vi "Send Settings.vi"(8 "error in":errorcluster, 11 "6700 in":refnum<class "6700.lvclass">) -> (0 "error out":errorcluster, 3 "6700 out":refnum<class "6700.lvclass">)   [LabVIEW 2018, in "6700.lvlib" / "6700.lvclass"]
uses:
  6700.lvclass
  6700.lvclass/6700.ctl
  <instrlib>/Agilent N6700 Series/Agilent N6700 Series.lvlib
  builds/Power_Supply.lvlibp/Power Supply.lvclass
  C:/Users/Ron.Dexter.LUMINARTECH/Desktop/builds/Power_Supply.lvlibp/Power Supply.lvclass
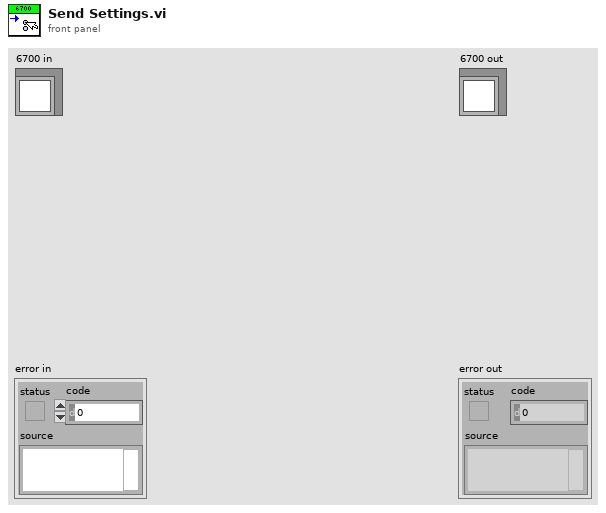
[diagram p1: front panel]
types:
  T1 = typedef "Power_Supply.lvlibp/Supply Settings.ctl" = cluster{"Voltage":dbl, "Current":dbl, "Output":bool}
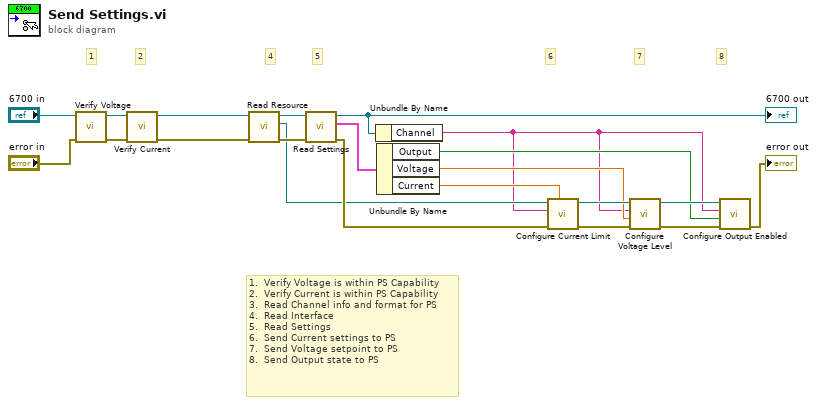
[diagram p0: block diagram]
diagram:
  # "1.  Verify Voltage is within PS Capability\n2.  Verify Current is within PS Capability\n3.  Read Channel info and format for PS\n4.  Read Interface\n5.  Read Settings\n6.  Send Current settings to PS\n7.  Send Voltage setpoint to PS\n8.  Send Output state to PS"
  # "8"
  # "7"
  # "6"
  # "5"
  # "4"
  # "2"
  # "1"
  n1 = call "Verify Voltage.vi"("error in"="error in", "6700 in"="6700 in") -> ("error out"=w19:errorcluster, "6700 out"=w21:refnum<class "6700.lvclass">)  [unwired: 8 in]
  n2 = call "Verify Current.vi"("error in"=w19, "6700 in"=w21) -> ("error out"=w4:errorcluster, "6700 out"=w3:refnum<class "6700.lvclass">)  [unwired: 8 in]
  n3 = call "Read Resource.vi"("error in"=w4, "Power Supply in"=w3) -> ("error out"=w6:errorcluster, "Resource"=w5:refnum<visa-resource-name>, "Power Supply out"=w7:refnum<class "6700.lvclass">)  [unwired: 7 in]
  n4 = call "Read Settings.vi"("error in (no error)"=w6, "Power Supply in"=w7) -> ("error out"=w11:errorcluster, "Settings"=w12:T1, "Power Supply out"=w1:refnum<class "6700.lvclass">)  [unwired: 7 in]
  "6700 out" <- w1
  n5 = Unbundle By Name(w1) -> ("Channel"=w2:string)
  n6 = Unbundle By Name(w12) -> ("Output"=w8:bool, "Voltage"=w9:dbl, "Current"=w10:dbl)
  n7 = call <instrlib>:"Configure Current Limit.vi"("Limit (0.0 amps)"=w10, "error in (no error)"=w11, "Channel Name (1)"=w2, "VISA resource name"=w5) -> ("error out"=w15:errorcluster, "VISA resource name out"=w14:refnum<visa-resource-name>)  [unwired: 6 in]
  n8 = call <instrlib>:"Configure Voltage Level.vi"("error in (no error)"=w15, "Level  (0.0 volts)"=w9, "Channel Name (1)"=w2, "VISA resource name"=w14) -> ("error out"=w17:errorcluster, "VISA resource name out"=w16:refnum<visa-resource-name>)  [unwired: 6 in]
  n9 = call <instrlib>:"Configure Output Enabled.vi"("error in (no error)"=w17, "Enable Output (False)"=w8, "Channel Name (1)"=w2, "VISA resource name"=w16) -> ("error out"=→"error out":errorcluster)  [unwired: 6 in, 1 out]
